vi "0 OCU - Networked.vi"() -> ()   [LabVIEW 2011]
doc: "This is the current implementation of the operator control unit (OCU) for small RC boat controlled by a host computer. The following features are currently implemented:\n- override control of the rudden angle and sail value by control interface or using keys\n- ability to add missions before and during a run\n- indicators for all relevant system status information\n\nAuthor: Jared Kirschner"
uses:
  2-Think/2 Typedefs/setpoints to boat.ctl
  2-Think/2 Typedefs/sail setpt.ctl
  2-Think/2 Typedefs/rudder angle.ctl
  2-Think/2 Typedefs/Velocity.ctl
  2-Think/2 Typedefs/apparent wind direction.ctl
  2-Think/2 Typedefs/apparent wind speed.ctl
  2-Think/2 Typedefs/apparent wind.ctl
  2-Think/2 Typedefs/heading.ctl
  2-Think/2 Typedefs/UTM Location.ctl
  2-Think/2 Typedefs/Which Boat.ctl
  2-Think/2 Typedefs/generalized sensor status.ctl
  2-Think/2 Typedefs/indicator LED.ctl
  2-Think/2 Typedefs/generalized actuator status.ctl
  0x2-OCU-Think Comm/0x2 Typedefs/Current Waypoint.ctl
  2-Think/2 Typedefs/robot velocity.ctl
  0x2-OCU-Think Comm/0x2 Typedefs/manual override.ctl
  0 Typedefs/Sail Position.ctl
  0 Typedefs/Rudder Position.ctl
  0 Typedefs/Apparent Wind Point of Sail.ctl
  0x2-OCU-Think Comm/0x2 Typedefs/ocuWaypoint.ctl
  0x2-OCU-Think Comm/0x2 Typedefs/Waypoints List.ctl
  2-Think/2 Classes/Waypoint/Waypoint.lvclass
  0 Typedefs/Mission Type Radio Buttons.ctl
  0x2-OCU-Think Comm/0x2 Typedefs/ocuMessage.ctl
  0x2-OCU-Think Comm/0x2 Typedefs/ocuCommands.ctl
  0x2-OCU-Think Comm/0x2 Typedefs/RIO-OCU update controls.ctl
  2-Think/2 Typedefs/rate of turn.ctl
  2-Think/2 Typedefs/pitch and roll.ctl
  2-Think/2 Typedefs/absolute wind direction.ctl
  2-Think/2 Typedefs/absolute wind speed.ctl
  2-Think/2 Typedefs/absolute water current vector.ctl
  2-Think/2 Typedefs/eStopCommand.ctl
  0x2-OCU-Think Comm/0x2 Classes/NetworkStreams/Reader/readType.ctl
  2-Think/2 Globals/2 Global.vi
  0x2-OCU-Think Comm/0x2 Classes/NetworkStreams/Reader/NetworkStreamReader.lvclass
  0x2-OCU-Think Comm/0x2 Classes/NetworkStreams/Writer/NetworkStreamWriter.lvclass
  2-Think/2 Classes/Mission/Mission.lvclass
panel:
  out "Rectangle":T1 {"Rotation" min=-90.0 max=90.0 step=1.0 format="%.2f"; "Left" scale=0.0..1024.0; "Right" scale=0.0..1024.0}
  out "Rudder Position":T2 scale=50.0..-50.0 scale format="%#.2g"
  out "Sail Position":T3
  out "Connected?":bool caption="Connection Status"
  in  "Location of THINK":string(combo)="127.0.0.1"
  in  "OVERRIDE SAIL?":bool
  in  "OVERRIDE RUDDER?":bool
  in  "E-Stop":bool
  out "Override Rudder Angle":dbl(slide) scale=-50.0..50.0
  out "Override Sail Value":dbl(slide) scale=0.0..1.0
  in  "OCU Tab Control":T4(tab)=enum."Before Mission: Define Mission"
  out "Connected":bool
  in  "Connect":bool
  out "Rudder Actuator Status":T5
  out "Sail Actuator Status":T5
  out "Wind Sensor Status":T7
  in  "Time(s)":dbl=300.0
  in  "Tolerance":dbl=0.5
  in  "Mission Type":T8
  in  "Map Path (relative)":path=path "locations/LPB Pool.png"
  out "# of Waypts":i32
  in  "Save Waypoints\nand PoI":bool
  in  "Save Image":bool
  out "Mission Map":T9(plugin-control)
  in  "Delete Last Waypoint":bool
  in  "Mission Def Filepath":path caption="MDF (Mission Definition File) path (leave blank for nothing)"
  in  "Globals":T10(tab)
  out "Which Boat Am I?":T11
  out "Battery Voltage":dbl
  out "Robot Heading":T12 format="%05.1f"
  out "Robot UTM Location":T13 {"North" format="%#_10f"; "East" format="%#_8f"}
  out "Overview Image":T9(plugin-control)
  out "Robot Velocity":T14
  out "Absolute Wind":T15
  out "Apparent Wind Direction":T16
  out "Apparent Wind Speed":T17
  out "Apparent Wind":T18
  out "Setpoints to boat":T19
  out "Sail Position":T20
  out "Rudder Angle":T21
  out "Current Waypoint":T22
  in  "Reset to start":bool
  out "Manual Override":T23
  out "Waypoints Array":T24[](array[typedef]) {"UTM Location"."North" format="%#_10f"; "UTM Location"."East" format="%#_8f"}
  out "Waypoints Object Array":T25
  out "Apparent Wind Direction\nPoint of Sail":T26 scale=0.0..360.0 scale format="%4d"
  # "TODO (Jason): finish this new representation"
  # "Manual Overide Control"
  # "Full Out = RIGHT"
  # "Out = UP"
  # "In = DOWN"
  # "Full In = LEFT"
  # "PORT"
  # "STARB"
  # "A"
  # "G"
  # "S"
  # "<--"
  # "D"
  # "-->"
  # "F"
  # "Map (required) and MDF (optional) are loaded on VI start.\nClick on map to add waypoints, pre-select attributes at right ->\nClick the appropriate buttons to save MDFs."
  # "TODO: check if the math for this is right :p"
  # "As Measured"
  # "From Planning Functions"
  # "Path Planning"
  # "(this is not a cluster because subitems\nare generated in parallel code)"
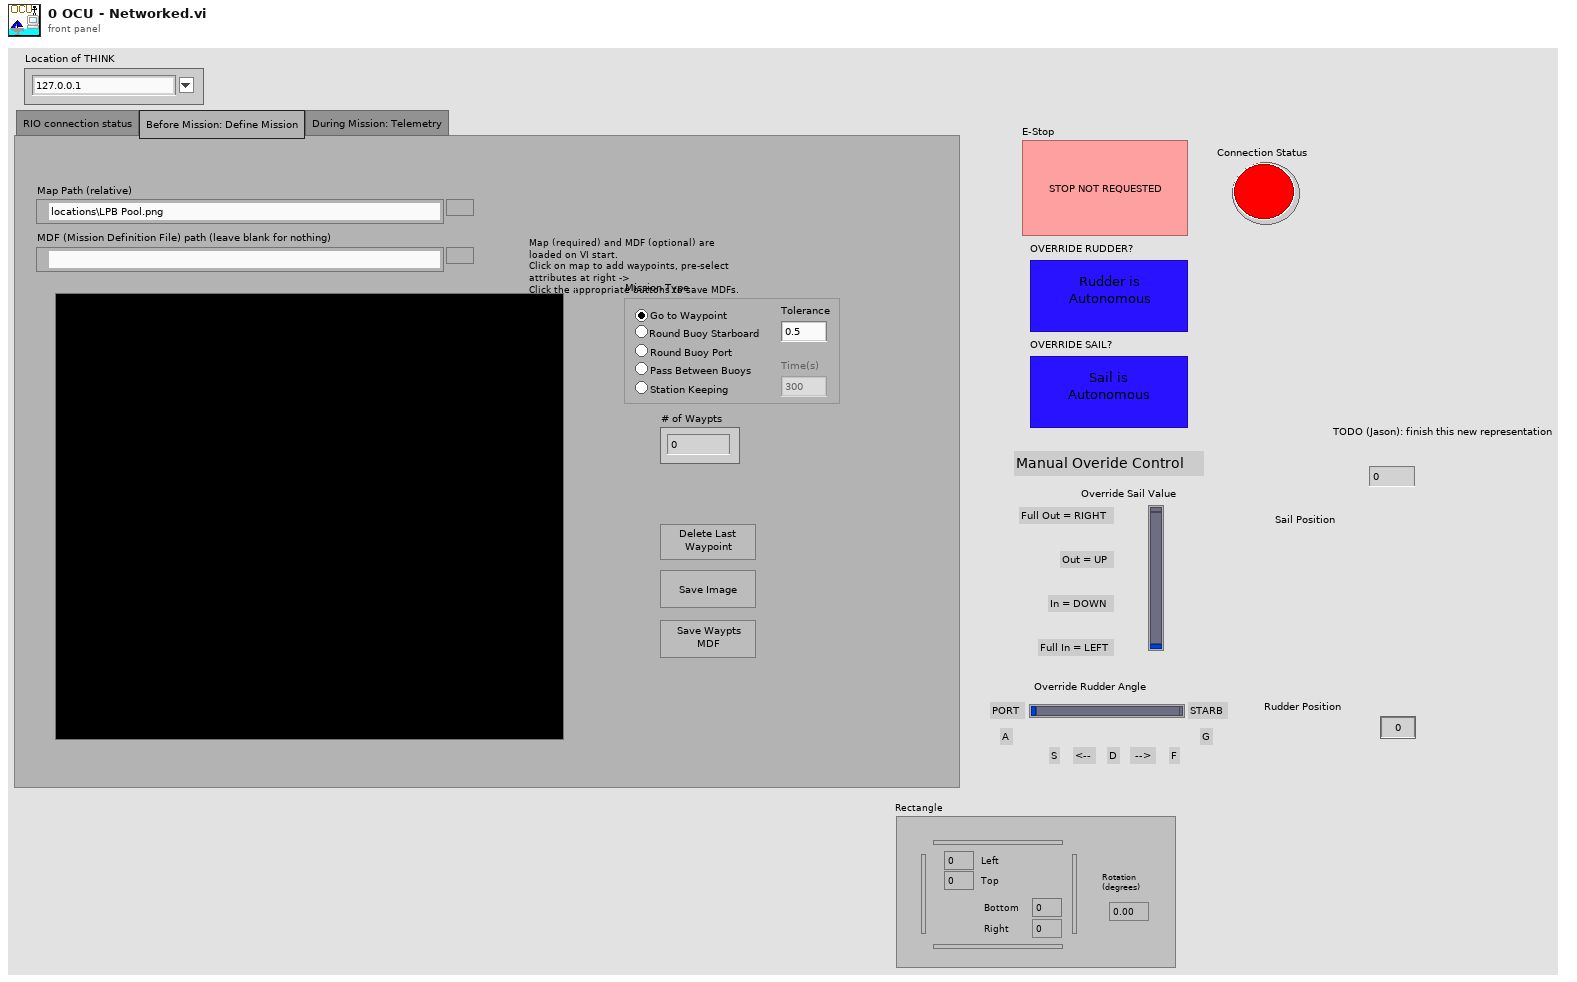
[diagram p1: front panel]
types:
  T1 = typedef "IMAQ Rectangle" = cluster{"Left":i32, "Top":i32, "Right":i32, "Bottom":i32, "Rotation":dbl}
  T2 = typedef "Rudder Position.ctl" = dbl
  T3 = typedef "Sail Position.ctl" = dbl
  T4 = enum32{"RIO connection status", "Before Mission: Define Mission", "During Mission: Telemetry"}
  T5 = typedef "generalized actuator status.ctl" = cluster{"Actuator Connected":T6}
  T6 = typedef "indicator LED.ctl" = bool
  T7 = typedef "generalized sensor status.ctl" = cluster{"Sensor Connected":T6, "Sensor Initialized":T6, "Sensor OK":T6, "Latest Error String":string, "GPS Lock":T6}
  T8 = typedef "Mission Type Radio Buttons.ctl" = enum32{"Go to Waypoint", "Round Buoy Starboard", "Round Buoy Port", "Pass Between Buoys", "Station Keeping"}
  T9 = typedef "IMAQ Image.ctl" = refnum<image>
  T10 = enum32{"How Am I", "Where Am I", "What's Around Me", "Path Planning"}
  T11 = typedef "Which Boat.ctl" = enum16{"Competition Boat", "Small RC", "Simulation"}
  T12 = typedef "heading.ctl" = dbl
  T13 = typedef "UTM Location.ctl" = cluster{"UTM Zone":dbl, "Hemisphere":enum16{"North", "South"}, "East":dbl, "North":dbl}
  T14 = typedef "robot velocity.ctl" = cluster{"East":dbl, "North":dbl}
  T15 = typedef "Velocity.ctl" = cluster{"East":dbl, "North":dbl}
  T16 = typedef "apparent wind direction.ctl" = dbl
  T17 = typedef "apparent wind speed.ctl" = dbl
  T18 = typedef "apparent wind.ctl" = cluster{"Toward Fore":dbl, "Toward Starboard":dbl}
  T19 = typedef "setpoints to boat.ctl" = cluster{"Sail Position":T20, "Rudder Angle":T21}
  T20 = typedef "sail setpt.ctl" = dbl
  T21 = typedef "rudder angle.ctl" = dbl
  T22 = typedef "Current Waypoint.ctl" = i32
  T23 = typedef "manual override.ctl" = cluster{"Override Active Rudder":bool, "Setpoints":T19, "Override Active Sail":bool}
  T24 = typedef "ocuWaypoint.ctl" = cluster{"Tolerance (m)":dbl, "UTM Location":T13}
  T25 = typedef "Waypoints List.ctl" = refnum<class "Waypoint.lvclass">[]
  T26 = typedef "Apparent Wind Point of Sail.ctl" = dbl
  T27 = typedef "RIO-OCU update controls.ctl" = cluster{"Sensor Status":T7, "Battery Voltage":dbl, "Rudder Actuator Status":T5, "Sail Actuator Status":T5, "Which Boat Am I?":T11, "Robot Velocity":T14, "Robot UTM Location":T13, "Robot\nHeading ":T12, "Robot\nRate of Turn":T28, "Robot Pitch/Roll":T29, "Apparent Wind":T18, "Apparent Wind\nSpeed":T17, "Apparent Wind\nDirection (º)":T16, "Absolute Wind":T15, "Absolute Wind\nDirection (º)":T30, "Absolute Wind\nSpeed":T31, "Absolute Water Current Vector":T32, "Rudder Angle":T21, "Sail Position":T20, "Manual Override Cluster":T23, "Setpoints to boat":T19, "Current Waypoint":T22, "Think freq.":dbl, "Sense freq.":dbl, "Act freq.":dbl, "E-stop freq.":dbl, "Network \nfreq.":dbl, "Network \nLoop Iterations":i64, "E-Stop":bool, "Serialized Waypoint Array":string}
  T28 = typedef "rate of turn.ctl" = dbl
  T29 = typedef "pitch and roll.ctl" = cluster{"Pitch":dbl, "Roll":dbl}
  T30 = typedef "absolute wind direction.ctl" = dbl
  T31 = typedef "absolute wind speed.ctl" = dbl
  T32 = typedef "absolute water current vector.ctl" = cluster{"Direction":T16, "Magnitude":T16}
  T33 = typedef "ocuMessage.ctl" = cluster{"OCU Command":T34, "Data":variant}
  T34 = typedef "ocuCommands.ctl" = enum16{"Pass", "Send override", "Add waypoint", "Delete waypoint", "Set waypoint number", "Stop", "Add Mission"}
  T35 = typedef "0-Image Descriptor.ctl" = cluster{"Upper-Left Corner Coordinates":T13, "Meters/Pixel":dbl}
  T36 = typedef "eStopCommand.ctl" = enum16{"Reset E-Stop", "Get E-Stop", "Set E-Stop"}
  T37 = typedef "NetworkStreamReader.lvclass/readType.ctl" = enum16{"Next in buffer", "Most current"}
  T38 = enum8{"Enabled", "Disabled", "Disabled and Grayed Out"}
  T39 = typedef "eventvkey.ctl" = enum16{"ASCII", "Enter", "Return", "Shift", "Ctrl", "Alt", "Cmd", "Opt", "Caps", "NumLock", "Clear", "Break", "Up", "Down", "Left", "Right", "Insert", "Delete", "Home", "End", "PageUp", "PageDown", "Escape", "Help", "Pause", "ScrollLock", "F1", "F2", "F3", "F4", "F5", "F6", "F7", "F8", "F9", "F10", "F11", "F12", "F13", "F14", "F15", "F16", "F17", "F18", "F19", "F20", "F21", "F22", "F23", "F24", "Play", "VolumeUp", "VolumeDown", "Mute", "Two Byte Char"}
  T40 = cluster{"Global Rectangle":i32[], "Contours":cluster{"Contour Type":u32, "ROI Type":u32, "Points":i32[]}[]}
  T41 = cluster{"Contour Type":u32, "ROI Type":u32, "Points":i32[]}[]
  T42 = cluster{"Contour Type":u32, "ROI Type":u32, "Points":i32[]}
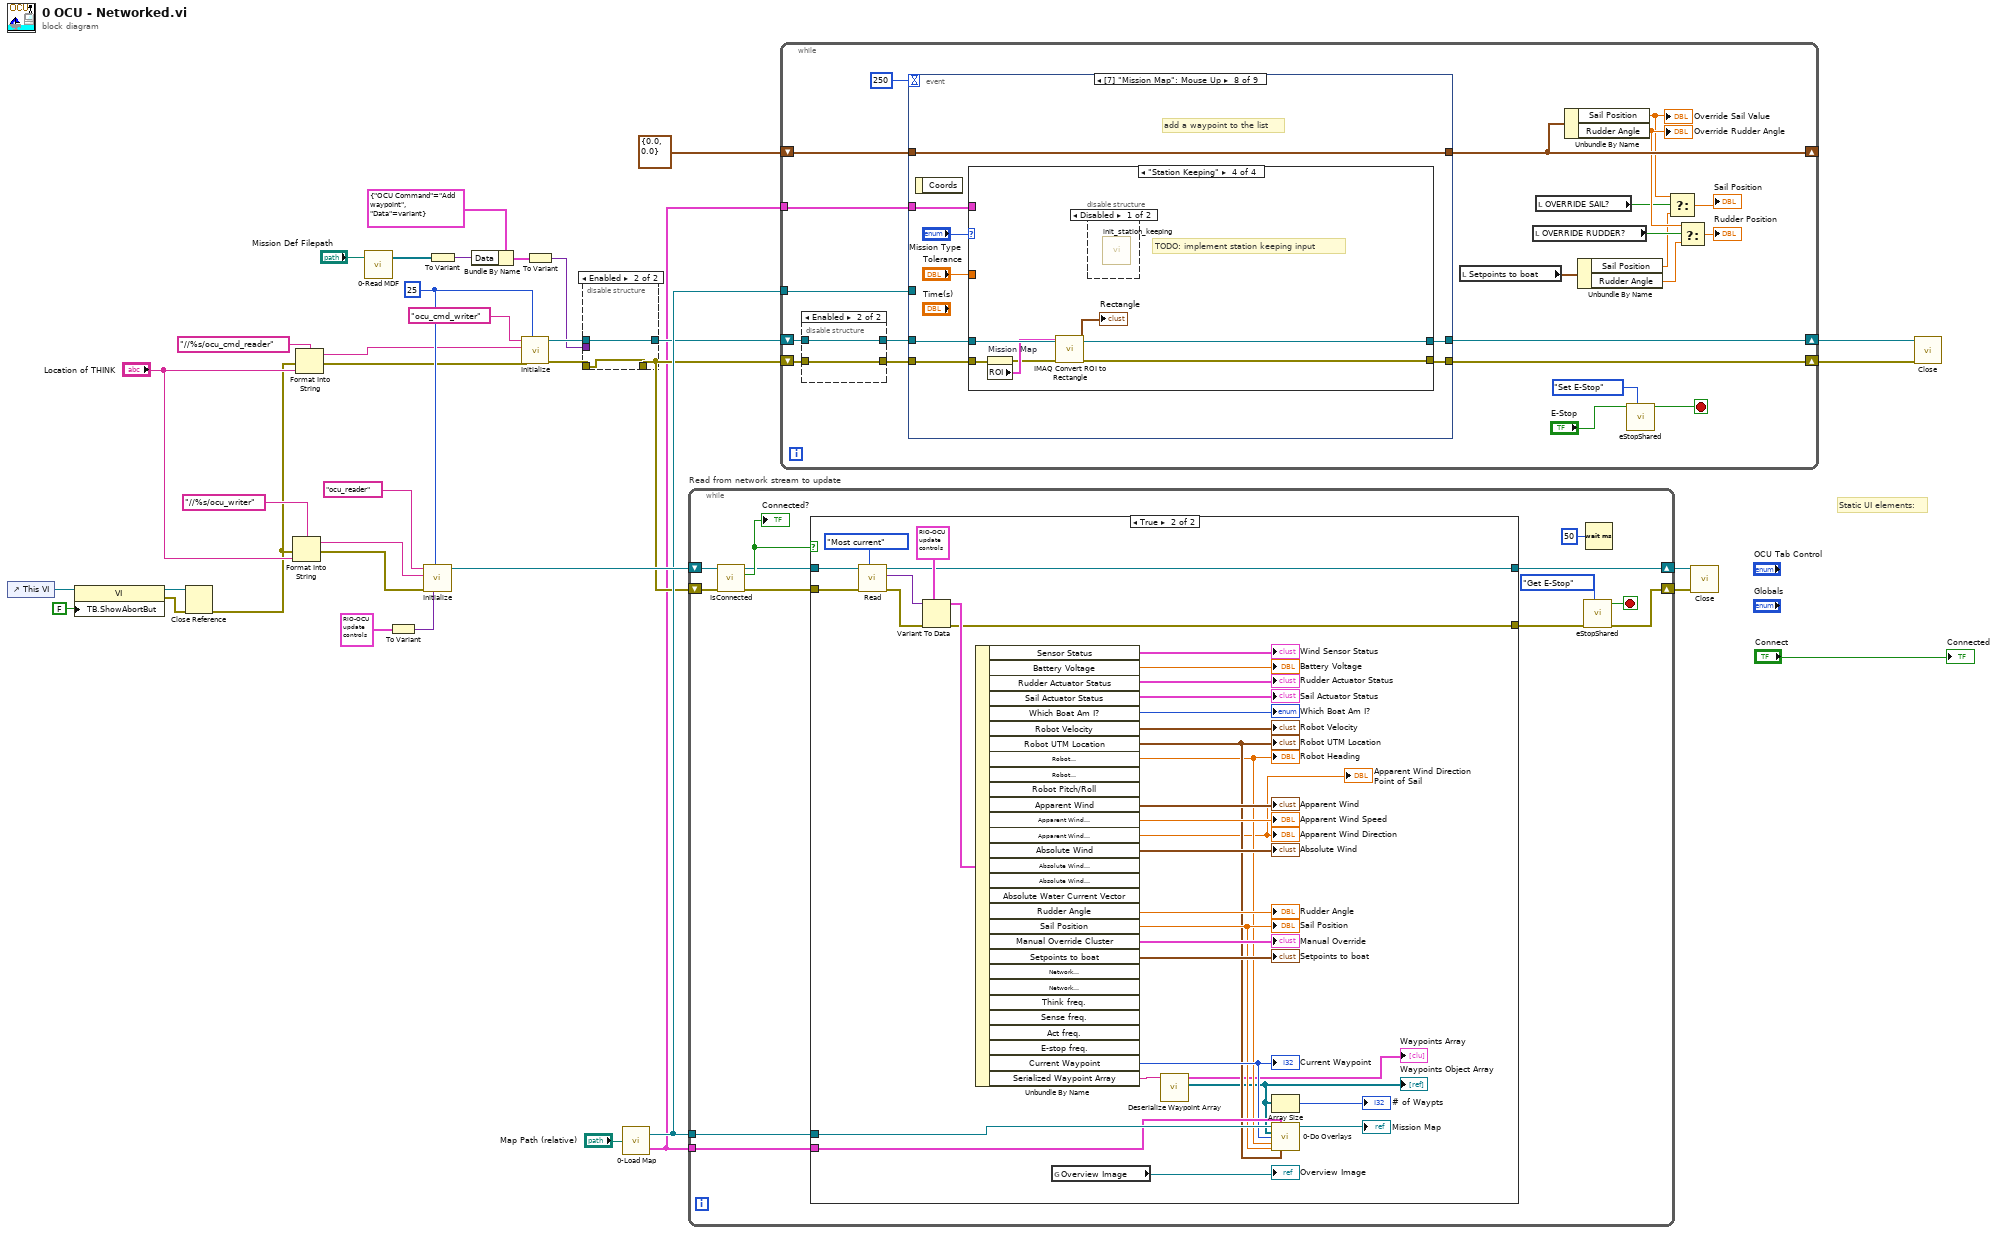
[diagram p0: block diagram]
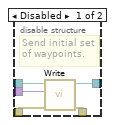
[diagram p2: hidden frame]
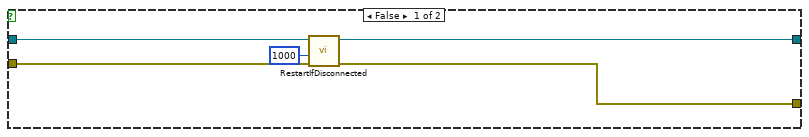
[diagram p3: hidden frame]
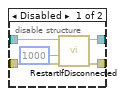
[diagram p4: hidden frame]
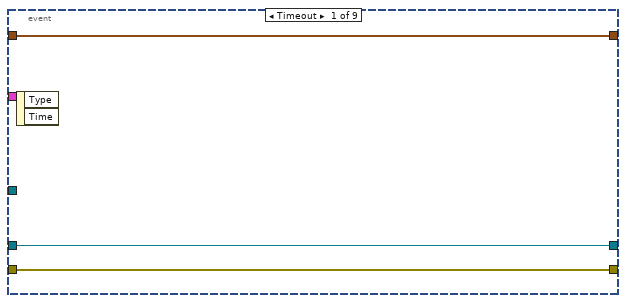
[diagram p5: hidden frame]
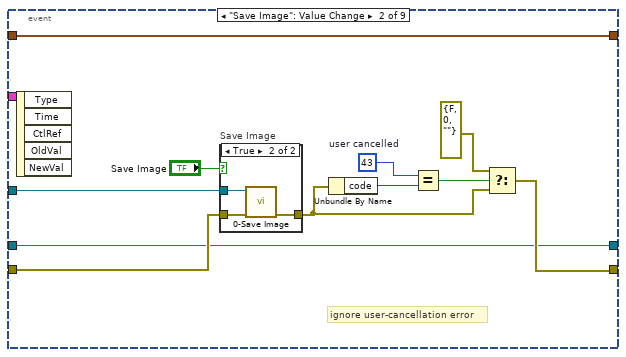
[diagram p6: hidden frame]
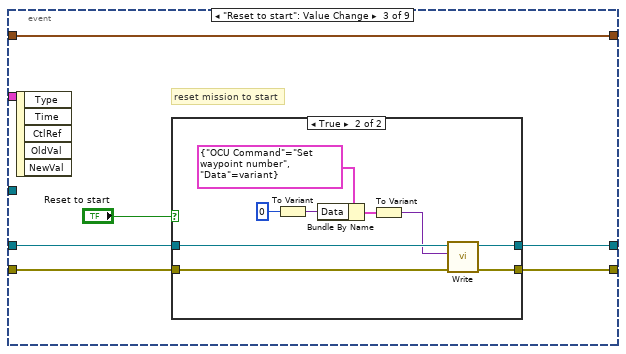
[diagram p8: hidden frame]
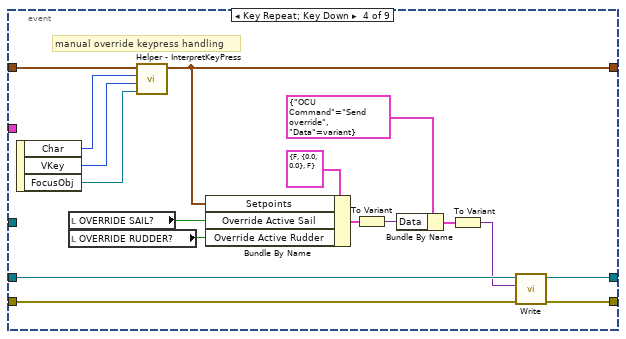
[diagram p10: hidden frame]
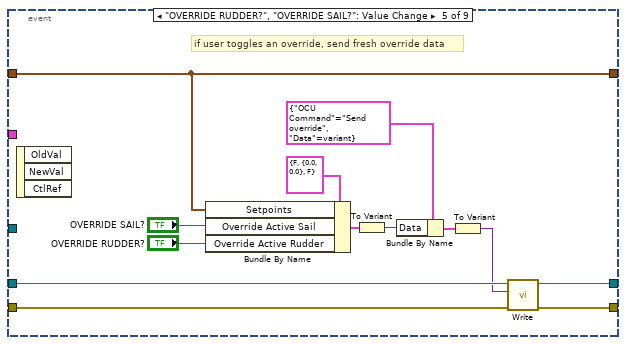
[diagram p11: hidden frame]
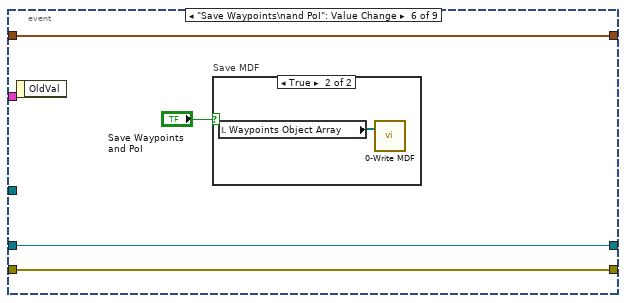
[diagram p12: hidden frame]
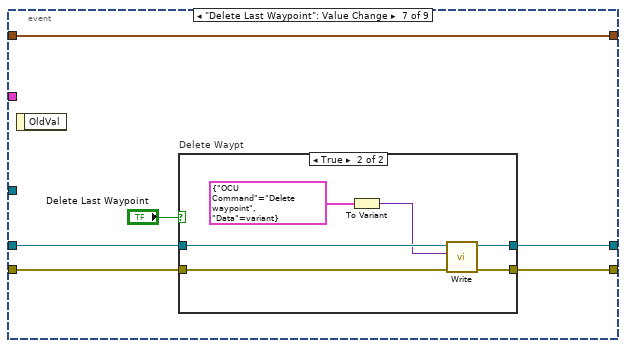
[diagram p14: hidden frame]
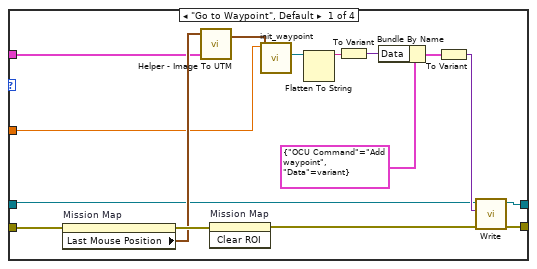
[diagram p16: hidden frame]
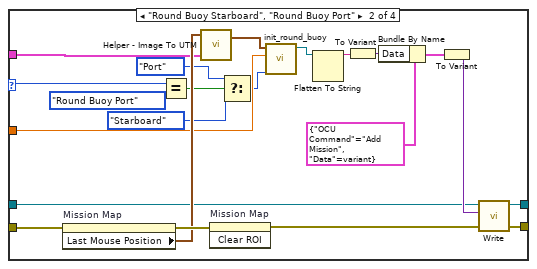
[diagram p17: hidden frame]
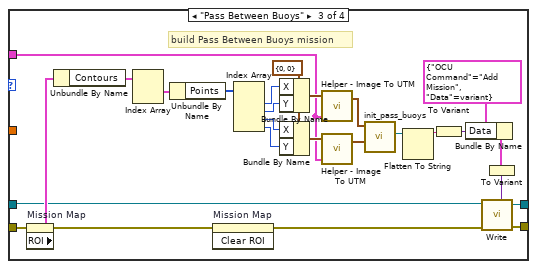
[diagram p18: hidden frame]
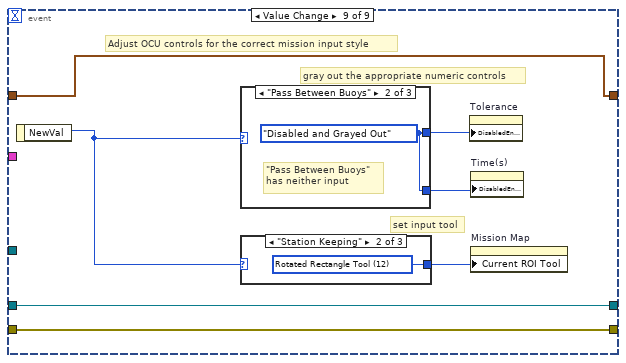
[diagram p20: hidden frame]
diagram:
  w32 = 25 ("writer buffer size")
  # "Static UI elements:"
  n1 = control-ref of="This VI"() -> (w13:refnum<vi>)
  n2 = property class="VI"(reference=w13, "TB.ShowAbortBut"=FALSE ("Tool Bar:Show Abort Button")) -> (reference out=w11:refnum<vi>, error out=w10:errorcluster)  [unwired: 1 in]
  n3 = Close Reference(reference=w11, error in (no error)=w10) -> (error out=w9:errorcluster)
  n4 = Format Into String(format string="//%s/ocu_writer", error in=w9, "Location of THINK") -> (resulting string=w3:string, error out=w7:errorcluster)  [unwired: 1 in]
  n5 = Format Into String(format string="//%s/ocu_cmd_reader", error in=w9, "Location of THINK") -> (resulting string=w1:string, error out=w8:errorcluster)  [unwired: 1 in]
  n6 = call "0-Read MDF.vi"("MDF file path"="Mission Def Filepath") -> ("Waypoints List"=w19:T25)  [unwired: 1 in, 1 out]
  n7 = To Variant(anything=T27 {"Sensor Status"={"Sensor Connected"=FALSE, "Sensor Initialized"=FALSE, "Sensor OK"=FALSE, "Latest Error String"="", "GPS Lock"=FALSE}, "Battery Voltage"=0.0, "Rudder Actuator Status"={"Actuator Connected"=FALSE}, "Sail Actuator Status"={"Actuator Connected"=FALSE}, "Which Boat Am I?"=enum."Competition Boat", "Robot Velocity"={"East"=0.0, "North"=0.0}, "Robot UTM Location"={"UTM Zone"=0.0, "Hemisphere"=enum."North", "East"=0.0, "North"=0.0}, "Robot\nHeading "=0.0, "Robot\nRate of Turn"=0.0, "Robot Pitch/Roll"={"Pitch"=0.0, "Roll"=0.0}, "Apparent Wind"={"Toward Fore"=0.0, "Toward Starboard"=0.0}, "Apparent Wind\nSpeed"=0.0, "Apparent Wind\nDirection (º)"=0.0, "Absolute Wind"={"East"=0.0, "North"=0.0}, "Absolute Wind\nDirection (º)"=0.0, "Absolute Wind\nSpeed"=0.0, "Absolute Water Current Vector"={"Direction"=0.0, "Magnitude"=0.0}, "Rudder Angle"=0.0, "Sail Position"=0.0, "Manual Override Cluster"={"Override Active Rudder"=FALSE, "Setpoints"={"Sail Position"=0.0, "Rudder Angle"=0.0}, "Override Active Sail"=FALSE}, "Setpoints to boat"={"Sail Position"=0.0, "Rudder Angle"=0.0}, "Current Waypoint"=0, "Think freq."=0.0, "Sense freq."=0.0, "Act freq."=0.0, "E-stop freq."=0.0, "Network \nfreq."=0.0, "Network \nLoop Iterations"=0, "E-Stop"=FALSE, "Serialized Waypoint Array"=""} ("RIO->OCU update data")) -> (Variant=w31:variant)
  n8 = call "Initialize.vi"("Default return"=w31, "reader buffer size"=w32, "error in (no error)"=w7, "writer url"=w3, "reader name"="ocu_reader" ("writer name")) -> ("NetworkStreamWriter out"=w33:refnum<class "NetworkStreamReader.lvclass">)  [unwired: 4 in, 2 out]
  n9 = To Variant(anything=w19) -> (Variant=w20:variant)
  n10 = Bundle By Name(cluster=T33 {"OCU Command"=enum."Add waypoint", "Data"=variant}, "Data"=w20) -> (w22:T33)
  n11 = call "Initialize.vi"("writer buffer size"=w32, "error in (no error)"=w8, "reader url"=w1, "writer name"="ocu_cmd_writer") -> ("error out"=w26:errorcluster, "NetworkStreamWriter out"=w27:refnum<class "NetworkStreamWriter.lvclass">)  [unwired: 5 in, 1 out]
  n12 = To Variant(anything=w22) -> (Variant=w21:variant)
  n13 = disable-structure shown="Enabled" {
    disable-tunnel: w27 -> [w42 w44]
    disable-tunnel: w26 -> [w41 w43]
    disable-tunnel: [w40 w43] -> w25
    disable-tunnel: [w39 w44] -> w24
    disable-tunnel: w21 -> [w38 _]
    frame Disabled {
      # "Send initial set\nof waypoints."
      n14 = call "Write.vi"("error in (no error)"=w41, "element"=w38, "NetworkStreamWriter in"=w42) -> ("error out"=w40:errorcluster, "NetworkStreamWriter out"=w39:refnum<class "NetworkStreamWriter.lvclass">)  [unwired: 6 in, 1 out]
    }
    frame Enabled {
    }
  }
  n15 = call "0-Load Map.vi"("Image Path"="Map Path (relative)") -> ("Image Out"=w28:T9, "Image Descriptor"=w5:T35)
  n16 = while "Read from network stream to update" {
    shift-right: [w57] -> w30
    shift-left: w33 -> [w52]
    shift-right: [w50] -> w29
    shift-left: w25 -> [w51]
    tunnel: w28 -> [w54]
    tunnel: w5 -> [w53]
    stop <- w55 stop-if-true
    n17 = call "IsConnected.vi"("error in (no error)"=w51, "NetworkStreamReader in"=w52) -> ("error out"=w46:errorcluster, "Connected?"=w48:bool, "NetworkStreamReader out"=w47:refnum<class "NetworkStreamReader.lvclass">)  [unwired: 7 in]
    "Connected?" <- w48
    n18 = case shown="True" w48 {
      tunnel: [w60 w92] -> w57
      tunnel: w54 -> [_ w77]
      tunnel: w53 -> [_ w74]
      tunnel: w47 -> [w62 w70]
      tunnel: w46 -> [w61 w69]
      tunnel: [w59 w68] -> w45
      frame False {
        n19 = call "RestartIfDisconnected.vi"("error in (no error)"=w61, "connection timeout"=1000, "NetworkStreamReader in"=w62) -> ("error out"=w59:errorcluster, "NetworkStreamReader out"=w60:refnum<class "NetworkStreamReader.lvclass">)  [unwired: 7 in]
      }
      frame True {
        n20 = call "Read.vi"("Read Type"=readType."Most current", "error in (no error)"=w69, "NetworkStreamReader in"=w70) -> ("error out"=w95:errorcluster, "element"=w94:variant, "NetworkStreamReader out"=w92:refnum<class "NetworkStreamReader.lvclass">)  [unwired: 4 in, 2 out]
        n21 = Variant To Data(error in=w95, type=T27 {"Sensor Status"={"Sensor Connected"=FALSE, "Sensor Initialized"=FALSE, "Sensor OK"=FALSE, "Latest Error String"="", "GPS Lock"=FALSE}, "Battery Voltage"=0.0, "Rudder Actuator Status"={"Actuator Connected"=FALSE}, "Sail Actuator Status"={"Actuator Connected"=FALSE}, "Which Boat Am I?"=enum."Competition Boat", "Robot Velocity"={"East"=0.0, "North"=0.0}, "Robot UTM Location"={"UTM Zone"=0.0, "Hemisphere"=enum."North", "East"=0.0, "North"=0.0}, "Robot\nHeading "=0.0, "Robot\nRate of Turn"=0.0, "Robot Pitch/Roll"={"Pitch"=0.0, "Roll"=0.0}, "Apparent Wind"={"Toward Fore"=0.0, "Toward Starboard"=0.0}, "Apparent Wind\nSpeed"=0.0, "Apparent Wind\nDirection (º)"=0.0, "Absolute Wind"={"East"=0.0, "North"=0.0}, "Absolute Wind\nDirection (º)"=0.0, "Absolute Wind\nSpeed"=0.0, "Absolute Water Current Vector"={"Direction"=0.0, "Magnitude"=0.0}, "Rudder Angle"=0.0, "Sail Position"=0.0, "Manual Override Cluster"={"Override Active Rudder"=FALSE, "Setpoints"={"Sail Position"=0.0, "Rudder Angle"=0.0}, "Override Active Sail"=FALSE}, "Setpoints to boat"={"Sail Position"=0.0, "Rudder Angle"=0.0}, "Current Waypoint"=0, "Think freq."=0.0, "Sense freq."=0.0, "Act freq."=0.0, "E-stop freq."=0.0, "Network \nfreq."=0.0, "Network \nLoop Iterations"=0, "E-Stop"=FALSE, "Serialized Waypoint Array"=""} ("RIO->OCU update data"), Variant=w94) -> (data=w91:T27, error out=w68:errorcluster)
        n22 = Unbundle By Name(w91) -> ("Sensor Status"=→"Wind Sensor Status":T7, "Battery Voltage"=→"Battery Voltage":dbl, "Rudder Actuator Status"=→"Rudder Actuator Status":T5, "Sail Actuator Status"=→"Sail Actuator Status":T5, "Which Boat Am I?"=→"Which Boat Am I?":T11, "Robot Velocity"=→"Robot Velocity":T14, "Robot UTM Location"=w71:T13, "Robot\nHeading"=w67:T12, "Apparent Wind"=→"Apparent Wind":T18, "Apparent Wind\nSpeed"=→"Apparent Wind Speed":T17, "Apparent Wind\nDirection (º)"=→"Apparent Wind Direction" →"Apparent Wind Direction\nPoint of Sail":T16, "Absolute Wind"=→"Absolute Wind":T15, "Rudder Angle"=→"Rudder Angle":T21, "Sail Position"=w72:T20, "Manual Override Cluster"=→"Manual Override":T23, "Setpoints to boat"=→"Setpoints to boat":T19, "Current Waypoint"=w73:T22, "Serialized Waypoint Array"=w66:string)  [unwired: 11 out]
        "Robot UTM Location" <- w71
        "Robot Heading" <- w67
        "Sail Position" <- w72
        "Current Waypoint" <- w73
        n23 = global read "2 Global.vi" "Overview Image"() -> (→"Overview Image":T9)
        n24 = call "Deserialize Waypoint Array.vi"("Serialized Waypoint Array"=w66) -> ("Waypoints Object Array"=w64:T25, "Waypoints Array"=→"Waypoints Array":T24[])  [unwired: 9 in]
        "Waypoints Object Array" <- w64
        n25 = Array Size(array=w64) -> (size(s)=→"# of Waypts":i32)
        n26 = call "0-Do Overlays.vi"("Image in"=w77, "Image Descriptor"=w74, "Waypoints List"=w64, "Current Waypoint #"=w73, "Heading"=w67, "Sail Position"=w72, "Robot UTM Location"=w71) -> ("Image out"=→"Mission Map":T9)  [unwired: 8 in]
      }
    }
    n27 = call "eStopShared.vi"("Command"=eStopCommand."Get E-Stop", "Error In"=w45) -> ("Error Out"=w50:errorcluster, "E-Stop Out"=w55:bool)  [unwired: 8 in]
    n28 = Wait (ms)(milliseconds to wait=u32 50 ("millisecond multiple")) -> ()  [unwired: 1 out]
  }
  n29 = while {
    shift-right: [w117] -> w14
    shift-left: w25 -> [w99]
    shift-right: [w111] -> _
    shift-left: T19 {"Sail Position"=0.0, "Rudder Angle"=0.0} ("Setpoints") -> [w119]
    shift-right: [w113] -> w15
    shift-left: w24 -> [w100]
    tunnel: w28 -> [w112]
    tunnel: w5 -> [w110]
    stop <- w116 stop-if-true
    n30 = disable-structure shown="Enabled" {
      disable-tunnel: w100 -> [w124 w126]
      disable-tunnel: w99 -> [w123 w125]
      disable-tunnel: [w122 w126] -> w98
      disable-tunnel: [w121 w125] -> w97
      frame Disabled {
        n31 = call "RestartIfDisconnected.vi"("error in (no error)"=w123, "connection timeout"=1000, "NetworkStreamWriter in"=w124) -> ("error out"=w121:errorcluster, "NetworkStreamWriter out"=w122:refnum<class "NetworkStreamWriter.lvclass">)  [unwired: 7 in]
      }
      frame Enabled {
      }
    }
    n32 = event shown="[7] \"Mission Map\": Mouse Up" {
      selector: _ -> [_ _ _ _ _ _ _ _ _]
      dyn-events: _ -> [_ _ _ _ _ _ _ _ _]
      timeout: 250 -> [_ _ _ _ _ _ _ _ _]
      tunnel: w119 -> [w129 w136 w150 w178 w181 w194 w201 w218 w288]
      tunnel: [w129 w136 w150 w174 w181 w194 w201 w218 w288] -> w111
      tunnel: w97 -> [w127 w134 w147 w171 w188 w193 w199 w217 w289]
      tunnel: [w127 w131 w145 w170 w187 w193 w197 w213 w289] -> w117
      tunnel: w98 -> [w128 w130 w148 w173 w190 w192 w200 w211 w290]
      tunnel: [w128 w130 w146 w172 w189 w192 w198 w212 w290] -> w113
      tunnel: w112 -> [_ w135 _ _ _ _ _ _ _]
      tunnel: w110 -> [_ _ _ _ _ _ _ w216 _]
      event Timeout {
        n33 = event-data() -> ()  [unwired: 1 in, 2 out]
      }
      event "Save Image": Value Change {
        w139 = 43  # user cancelled
        # "ignore user-cancellation error"
        n34 = event-data() -> ()  [unwired: 1 in, 5 out]
        n35 = case "Save Image" shown="True" "Save Image" {
          tunnel: w134 -> [w141 w144]
          tunnel: [w141 w143] -> w133
          tunnel: w135 -> [_ w142]
          frame False {
          }
          frame True {
            n36 = call "0-Save Image.vi"("Error In"=w144, "Image in"=w142) -> ("Error Out"=w143:errorcluster)  [unwired: 9 in]
          }
        }
        n37 = Unbundle By Name(w133) -> ("code"=w140:i32)
        n38 = Equal?(x=w139, y=w140) -> (x = y?=w138:bool)
        n39 = Select(t=errorcluster {"status"=FALSE, "code"=0, "source"=""}, s=w138, f=w133) -> (s? t:f=w131:errorcluster)
      }
      event "Reset to start": Value Change {
        # "reset mission to start"
        n40 = event-data() -> ()  [unwired: 1 in, 5 out]
        n41 = case shown="True" "Reset to start" {
          tunnel: w148 -> [w152 w158]
          tunnel: w147 -> [w151 w159]
          tunnel: [w152 w161] -> w146
          tunnel: [w151 w160] -> w145
          frame False {
          }
          frame True {
            n42 = To Variant(anything=T22 0 ("Current Waypoint")) -> (Variant=w156:variant)
            n43 = Bundle By Name(cluster=T33 {"OCU Command"=enum."Set waypoint number", "Data"=variant}, "Data"=w156) -> (w154:T33)
            n44 = To Variant(anything=w154) -> (Variant=w153:variant)
            n45 = call "Write.vi"("error in (no error)"=w159, "element"=w153, "NetworkStreamWriter in"=w158) -> ("error out"=w160:errorcluster, "NetworkStreamWriter out"=w161:refnum<class "NetworkStreamWriter.lvclass">)  [unwired: 6 in, 1 out]
          }
        }
      }
      event Key Repeat; Key Down {
        # "manual override keypress handling"
        n46 = event-data() -> ("Char"=w177:i16, "VKey"=w176:T39, "FocusObj"=w162:refnum<vi>)  [unwired: 1 in]
        n47 = local read "OVERRIDE SAIL?"() -> (w163:bool)
        n48 = local read "OVERRIDE RUDDER?"() -> (w164:bool)
        n49 = call "Helper - InterpretKeyPress.vi"("FocusObj"=w162, "VKey"=w176, "Char"=w177, "Command In"=w178) -> ("Command Out"=w174:T19)  [unwired: 7 in]
        n50 = Bundle By Name(cluster=T23 {"Override Active Rudder"=FALSE, "Setpoints"={"Sail Position"=0.0, "Rudder Angle"=0.0}, "Override Active Sail"=FALSE} ("Manual Override Cluster"), "Setpoints"=w174, "Override Active Sail"=w163, "Override Active Rudder"=w164) -> (w166:T23)
        n51 = To Variant(anything=w166) -> (Variant=w169:variant)
        n52 = Bundle By Name(cluster=T33 {"OCU Command"=enum."Send override", "Data"=variant}, "Data"=w169) -> (w168:T33)
        n53 = To Variant(anything=w168) -> (Variant=w165:variant)
        n54 = call "Write.vi"("error in (no error)"=w171, "element"=w165, "NetworkStreamWriter in"=w173) -> ("error out"=w170:errorcluster, "NetworkStreamWriter out"=w172:refnum<class "NetworkStreamWriter.lvclass">)  [unwired: 6 in, 1 out]
      }
      event "OVERRIDE RUDDER?", "OVERRIDE SAIL?": Value Change {
        # "if user toggles an override, send fresh override data"
        n55 = event-data() -> ()  [unwired: 1 in, 3 out]
        n56 = Bundle By Name(cluster=T23 {"Override Active Rudder"=FALSE, "Setpoints"={"Sail Position"=0.0, "Rudder Angle"=0.0}, "Override Active Sail"=FALSE} ("Manual Override Cluster"), "Setpoints"=w181, "Override Active Sail"="OVERRIDE SAIL?", "Override Active Rudder"="OVERRIDE RUDDER?") -> (w183:T23)
        n57 = To Variant(anything=w183) -> (Variant=w186:variant)
        n58 = Bundle By Name(cluster=T33 {"OCU Command"=enum."Send override", "Data"=variant}, "Data"=w186) -> (w185:T33)
        n59 = To Variant(anything=w185) -> (Variant=w182:variant)
        n60 = call "Write.vi"("error in (no error)"=w188, "element"=w182, "NetworkStreamWriter in"=w190) -> ("error out"=w187:errorcluster, "NetworkStreamWriter out"=w189:refnum<class "NetworkStreamWriter.lvclass">)  [unwired: 6 in, 1 out]
      }
      event "Save Waypoints\nand PoI": Value Change {
        n61 = event-data() -> ()  [unwired: 1 in, 1 out]
        n62 = case "Save MDF" shown="True" "Save Waypoints\nand PoI" {
          frame False {
          }
          frame True {
            n63 = local read "Waypoints Object Array"() -> (w196:T25)
            n64 = call "0-Write MDF.vi"("Waypoints List"=w196) -> ()  [unwired: 2 in, 1 out]
          }
        }
      }
      event "Delete Last Waypoint": Value Change {
        n65 = event-data() -> ()  [unwired: 1 in, 1 out]
        n66 = case "Delete Waypt" shown="True" "Delete Last Waypoint" {
          tunnel: w200 -> [w204 w210]
          tunnel: w199 -> [w203 w209]
          tunnel: [w204 w208] -> w198
          tunnel: [w203 w207] -> w197
          frame False {
          }
          frame True {
            n67 = To Variant(anything=T33 {"OCU Command"=enum."Delete waypoint", "Data"=variant}) -> (Variant=w205:variant)
            n68 = call "Write.vi"("error in (no error)"=w209, "element"=w205, "NetworkStreamWriter in"=w210) -> ("error out"=w207:errorcluster, "NetworkStreamWriter out"=w208:refnum<class "NetworkStreamWriter.lvclass">)  [unwired: 6 in, 1 out]
          }
        }
      }
      event "Mission Map": Mouse Up {
        # "add a waypoint to the list"
        n69 = event-data() -> ()  [unwired: 1 in, 1 out]
        n70 = case shown="\"Station Keeping\"" "Mission Type" {
          selector: "Mission Type" -> [_ w245 _ _]
          tunnel: w217 -> [w232 w253 w281 w286]
          tunnel: [w224 w250 w259 w282] -> w213
          tunnel: w216 -> [w229 w249 w256 _]
          tunnel: "Tolerance" -> [w225 w246 _ _]
          tunnel: [w222 w238 w262 w287] -> w212
          tunnel: w211 -> [w219 w235 w263 w287]
          frame "Go to Waypoint", Default {
            n71 = property on="Mission Map" class="ImageControl"(error in=w232) -> (error out=w234:errorcluster, "Last Mouse Position"=w233:cluster{"X":i32, "Y":i32})  [unwired: 1 in, 1 out]
            n72 = call "Helper - Image To UTM.vi"("Image Descriptor"=w229, "Pixel Coordinates"=w233) -> ("UTM Location"=w228:T13)  [unwired: 1 in, 1 out]
            n73 = invoke on="Mission Map" class="ImageControl" method="Clear ROI"(error in=w234) -> (error out=w223:errorcluster)  [unwired: 2 in, 2 out]
            n74 = call "init_waypoint.vi"("Coords"=w228, "Tolerance (m)"=w225) -> ("Waypoint Out"=w226:refnum<class "Waypoint.lvclass">)  [unwired: 9 in]
            n75 = Flatten To String(anything=w226) -> (data string=w227:string)  [unwired: 3 in, 2 out]
            n76 = To Variant(anything=w227) -> (Variant=w230:variant)
            n77 = Bundle By Name(cluster=T33 {"OCU Command"=enum."Add waypoint", "Data"=variant}, "Data"=w230) -> (w221:T33)
            n78 = To Variant(anything=w221) -> (Variant=w220:variant)
            n79 = call "Write.vi"("error in (no error)"=w223, "element"=w220, "NetworkStreamWriter in"=w219) -> ("error out"=w224:errorcluster, "NetworkStreamWriter out"=w222:refnum<class "NetworkStreamWriter.lvclass">)  [unwired: 6 in, 1 out]
          }
          frame "Round Buoy Starboard", "Round Buoy Port" {
            n80 = property on="Mission Map" class="ImageControl"(error in=w253) -> (error out=w255:errorcluster, "Last Mouse Position"=w254:cluster{"X":i32, "Y":i32})  [unwired: 1 in, 1 out]
            n81 = Equal?(x=w245, y=Mission_Type_Radio_Buttons."Round Buoy Port" ("Mission Type 2")) -> (x = y?=w240:bool)
            n82 = call "Helper - Image To UTM.vi"("Image Descriptor"=w249, "Pixel Coordinates"=w254) -> ("UTM Location"=w247:T13)  [unwired: 1 in, 1 out]
            n83 = invoke on="Mission Map" class="ImageControl" method="Clear ROI"(error in=w255) -> (error out=w250:errorcluster)  [unwired: 2 in, 2 out]
            n84 = Select(t=enum16{"Starboard", "Port"}."Port" ("Round side?"), s=w240, f=enum16{"Starboard", "Port"}."Starboard" ("Round side?")) -> (s? t:f=w241:enum16{"Starboard", "Port"})
            n85 = call "init_round_buoy.vi"("Round side?"=w241, "Tolerance (m)"=w246, "Buoy to Round"=w247) -> ("Mission out"=w239:refnum<class "Mission.lvclass">)  [unwired: 8 in]
            n86 = Flatten To String(anything=w239) -> (data string=w248:string)  [unwired: 3 in, 2 out]
            n87 = To Variant(anything=w248) -> (Variant=w251:variant)
            n88 = Bundle By Name(cluster=T33 {"OCU Command"=enum."Add Mission", "Data"=variant}, "Data"=w251) -> (w236:T33)
            n89 = To Variant(anything=w236) -> (Variant=w237:variant)
            n90 = call "Write.vi"("element"=w237, "NetworkStreamWriter in"=w235) -> ("NetworkStreamWriter out"=w238:refnum<class "NetworkStreamWriter.lvclass">)  [unwired: 7 in, 2 out]
          }
          frame "Pass Between Buoys" {
            w274 = cluster{"X":i32, "Y":i32} {"X"=0, "Y"=0} ("Pixel Coordinates")
            # "build Pass Between Buoys mission"
            n91 = property on="Mission Map" class="ImageControl"(error in=w281) -> (error out=w260:errorcluster, "ROI"=w280:T40)  [unwired: 1 in, 1 out]
            n92 = Unbundle By Name(w280) -> ("Contours"=w279:T41)
            n93 = Index Array(array=w279) -> (element #1=w278:T42)  [unwired: 2 in, 1 out]
            n94 = Unbundle By Name(w278) -> ("Points"=w276:i32[])
            n95 = invoke on="Mission Map" class="ImageControl" method="Clear ROI"(error in=w260) -> (error out=w261:errorcluster)  [unwired: 2 in, 2 out]
            n96 = Index Array(array=w276) -> (element #1=w273:i32, element #2=w272:i32, element #3=w271:i32, element #4=w270:i32)  [unwired: 4 in]
            n97 = Bundle By Name(cluster=w274, "X"=w273, "Y"=w272) -> (w277:cluster{"X":i32, "Y":i32})
            n98 = Bundle By Name(cluster=w274, "X"=w271, "Y"=w270) -> (w275:cluster{"X":i32, "Y":i32})
            n99 = call "Helper - Image To UTM.vi"("Image Descriptor"=w256, "Pixel Coordinates"=w277) -> ("UTM Location"=w269:T13)  [unwired: 1 in, 1 out]
            n100 = call "Helper - Image To UTM.vi"("Image Descriptor"=w256, "Pixel Coordinates"=w275) -> ("UTM Location"=w268:T13)  [unwired: 1 in, 1 out]
            n101 = call "init_pass_buoys.vi"("Buoy Pass 2"=w268, "Buoy Pass 1"=w269) -> ("Mission.lvclass"=w257:refnum<class "Mission.lvclass">)  [unwired: 9 in]
            n102 = Flatten To String(anything=w257) -> (data string=w265:string)  [unwired: 3 in, 2 out]
            n103 = To Variant(anything=w265) -> (Variant=w266:variant)
            n104 = Bundle By Name(cluster=T33 {"OCU Command"=enum."Add Mission", "Data"=variant}, "Data"=w266) -> (w264:T33)
            n105 = To Variant(anything=w264) -> (Variant=w258:variant)
            n106 = call "Write.vi"("error in (no error)"=w261, "element"=w258, "NetworkStreamWriter in"=w263) -> ("error out"=w259:errorcluster, "NetworkStreamWriter out"=w262:refnum<class "NetworkStreamWriter.lvclass">)  [unwired: 6 in, 1 out]
          }
          frame "Station Keeping" {
            # "TODO: implement station keeping input"
            n107 = property on="Mission Map" class="ImageControl"(error in=w286) -> (error out=w283:errorcluster, "ROI"=w284:T40)  [unwired: 1 in, 1 out]
            n108 = call "IMAQ Convert ROI to Rectangle"("error in (no error)"=w283, "ROI Descriptor"=w284) -> ("error out"=w282:errorcluster, "Rectangle"=→"Rectangle":T1)  [unwired: 7 in]
            n109 = disable-structure shown="Disabled" {
              frame Disabled {
                n110 = call "init_station_keeping.vi"() -> ()  [unwired: 11 in, 1 out]
              }
              frame Enabled {
              }
            }
          }
        }
      }
      event Value Change {
        # "gray out the appropriate numeric controls"
        # "set input tool"
        # "Adjust OCU controls for the correct mission input style"
        n111 = event-data() -> ("NewVal"=w293:T8)  [unwired: 1 in]
        n112 = case shown="\"Pass Between Buoys\"" w293 {
          tunnel: [T38."Enabled" ("Disabled") w297 T38."Disabled and Grayed Out" ("Disabled")] -> w292
          tunnel: [T38."Disabled and Grayed Out" ("Disabled") w297 T38."Enabled" ("Disabled")] -> w291
          frame "Go to Waypoint", Default {
          }
          frame "Pass Between Buoys" {
            w297 = T38."Disabled and Grayed Out" ("Disabled")
            # "\"Pass Between Buoys\"\nhas neither input"
          }
          frame "Station Keeping" {
          }
        }
        n113 = case shown="\"Station Keeping\"" w293 {
          tunnel: [w300 w301 w302] -> w294
          frame "Go to Waypoint", Default {
            w300 = u32 1 items=["Zoom Tool"=8, "Selection Tool"=0, "Pan Tool"=9, "Point Tool"=1, "Line Tool"=2, "Rectangle Tool"=3, "Rotated Rectangle Tool"=12, "Polyline Tool"=10, "Polygon Tool"=5, "Freehand Tool"=11, "Closed Freehand Tool"=6, "Ellipse Tool"=4, "Annulus Tool"=7] ("Current ROI Tool")
          }
          frame "Station Keeping" {
            w301 = u32 12 items=["Zoom Tool"=8, "Selection Tool"=0, "Pan Tool"=9, "Point Tool"=1, "Line Tool"=2, "Rectangle Tool"=3, "Rotated Rectangle Tool"=12, "Polyline Tool"=10, "Polygon Tool"=5, "Freehand Tool"=11, "Closed Freehand Tool"=6, "Ellipse Tool"=4, "Annulus Tool"=7] ("Current ROI Tool")
          }
          frame "Pass Between Buoys" {
            w302 = u32 2 items=["Zoom Tool"=8, "Selection Tool"=0, "Pan Tool"=9, "Point Tool"=1, "Line Tool"=2, "Rectangle Tool"=3, "Rotated Rectangle Tool"=12, "Polyline Tool"=10, "Polygon Tool"=5, "Freehand Tool"=11, "Closed Freehand Tool"=6, "Ellipse Tool"=4, "Annulus Tool"=7] ("Current ROI Tool")
          }
        }
        n114 = property on="Tolerance" class="DigNum (strict)"("DisabledEnum"=w292) -> ()  [unwired: 2 in, 2 out]
        n115 = property on="Time(s)" class="DigNum (strict)"("DisabledEnum"=w291) -> ()  [unwired: 2 in, 2 out]
        n116 = property on="Mission Map" class="ImageControl"("Current ROI Tool"=w294) -> ()  [unwired: 2 in, 2 out]
      }
    }
    n117 = local read "Setpoints to boat"() -> (w103:T19)
    n118 = local read "OVERRIDE RUDDER?"() -> (w109:bool)
    n119 = local read "OVERRIDE SAIL?"() -> (w104:bool)
    n120 = Unbundle By Name(w111) -> ("Sail Position"=w106:T20, "Rudder Angle"=w107:T21)
    "Override Sail Value" <- w106
    "Override Rudder Angle" <- w107
    n121 = Unbundle By Name(w103) -> ("Sail Position"=w102:T20, "Rudder Angle"=w101:T21)
    n122 = call "eStopShared.vi"("Command"=eStopCommand."Set E-Stop", "E-Stop"="E-Stop") -> ("E-Stop Out"=w116:bool)  [unwired: 8 in, 1 out]
    n123 = Select(t=w106, s=w104, f=w102) -> (s? t:f=→"Sail Position":T20)
    n124 = Select(t=w107, s=w109, f=w101) -> (s? t:f=→"Rudder Position":T21)
  }
  n125 = call "Close.vi"("error in (no error)"=w29, "NetworkStreamReader in"=w30) -> ()  [unwired: 8 in, 2 out]
  n126 = call "Close.vi"("error in (no error)"=w14, "NetworkStreamWriter in"=w15) -> ()  [unwired: 8 in, 2 out]
  "Connected" <- "Connect"
